vi "Backup - Acquisition Settings Dialog.vi"(8 "error in (no error)":errorcluster, 11 "Channels in":T1[](array[typedef])) -> (0 "error out":errorcluster, 3 "Channels out":T1[](array[typedef]))   [LabVIEW 2021]
uses:
  Task Cluster (with Add Remove Buttons).ctl
  DAQ/DAQ.lvlib
  Channel Cluster.ctl
panel:
  in  "Cancel Button":bool
  in  "OK Button":bool
  in  "Channel List":T2={"Add Button"=FALSE, "Remove Button"=FALSE, "DAQmx Task"="Mod3AI0-Temp", "Radio Buttons"=enum."Read"}
  # "DAQmx Global Channel"
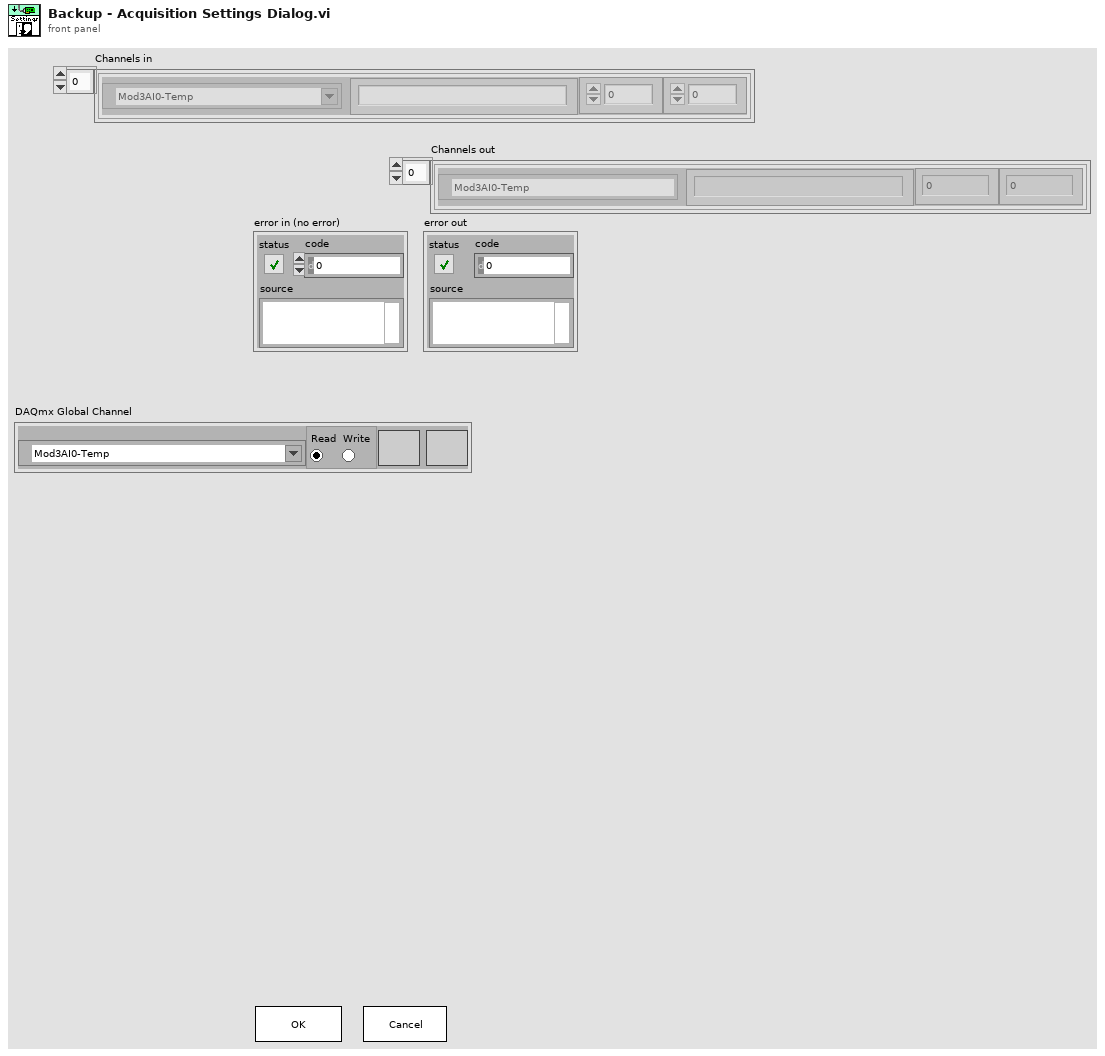
[diagram p1: front panel]
types:
  T1 = typedef "DAQ.lvlib/Channel Cluster.ctl" = cluster{"DAQmx Global Channel":refnum<k21>, "Tag Name":string, "Min Input":dbl, "Max Input":dbl}
  T2 = typedef "DAQ.lvlib/Task Cluster (with Add Remove Buttons).ctl" = cluster{"Add Button":bool, "Remove Button":bool, "DAQmx Task":refnum<k21>, "Radio Buttons":enum32{"Read", "Write"}}
  T3 = typedef "DAQ.lvlib/Channel Cluster (with Add Remove Buttons).ctl" = cluster{"Add Button":bool, "Remove Button":bool, "DAQmx Global Channel":refnum<k21>, "Tag Name":string, "Min Input":dbl, "Max Input":dbl}
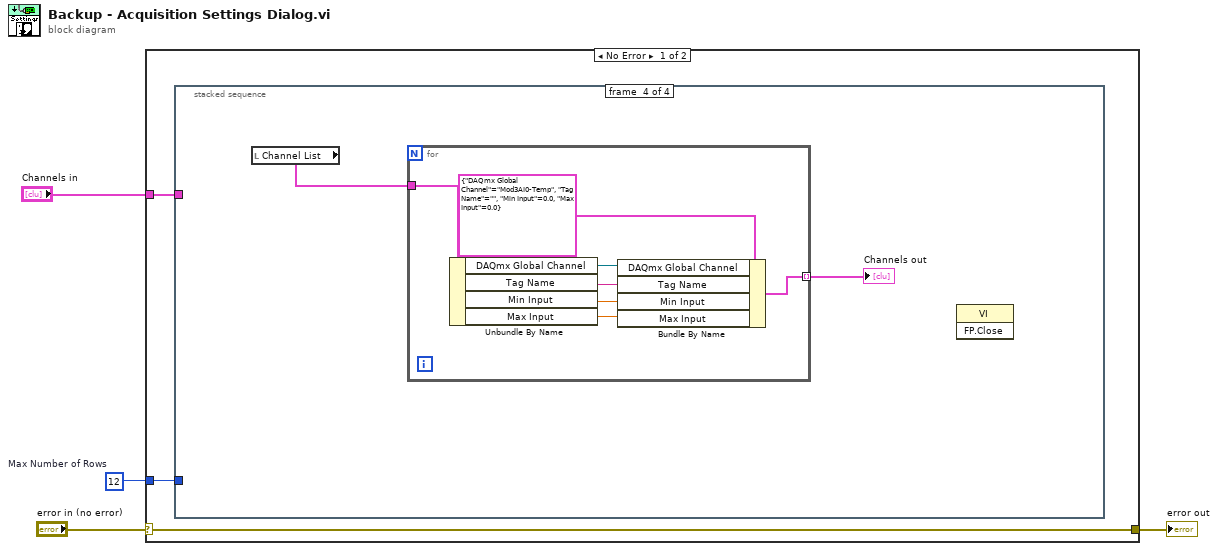
[diagram p0: block diagram]
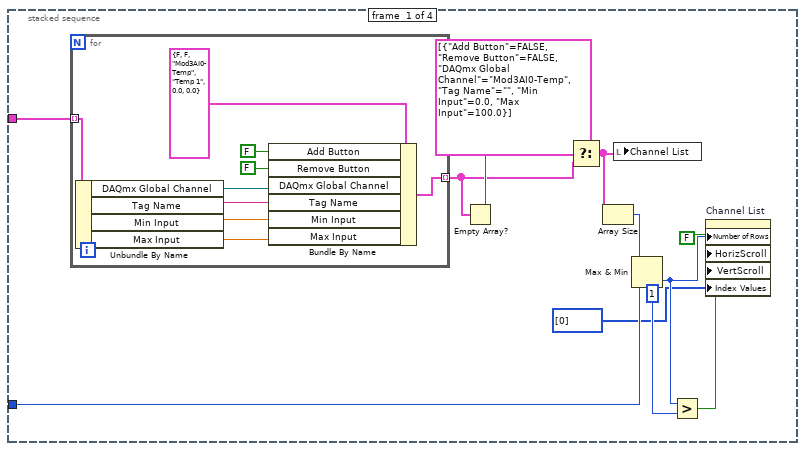
[diagram p2: hidden frame]
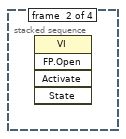
[diagram p3: hidden frame]
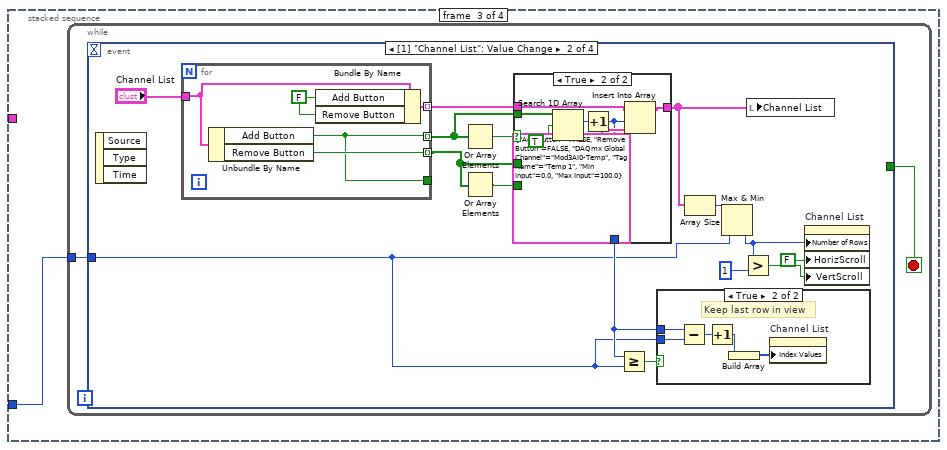
[diagram p4: hidden frame]
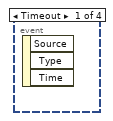
[diagram p5: hidden frame]
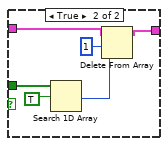
[diagram p8: hidden frame]
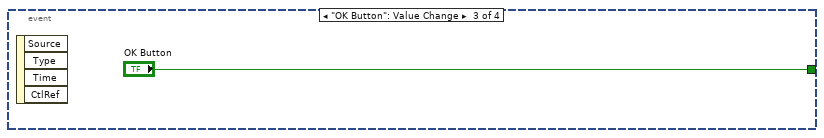
[diagram p9: hidden frame]
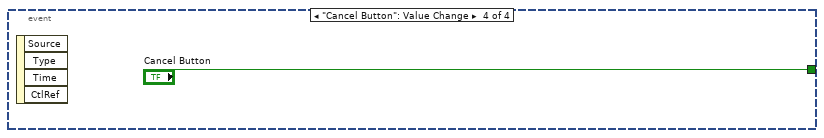
[diagram p10: hidden frame]
diagram:
  w1 = u32 12  # Max Number of Rows
  n1 = case shown="No Error" "error in (no error)" {
    selector: "error in (no error)" -> [w7 w86]
    tunnel: [w7 w86] -> w3
    tunnel: "Channels in" -> [w6 _]
    tunnel: w1 -> [w5 _]
    frame No Error {
      n2 = stacked-sequence {
        tunnel: w6 -> [w19 _ _ _]
        tunnel: w5 -> [w13 _ w29 _]
        frame #0 {
          n3 = for {
            tunnel: w19 -> [w28] mode=indexing
            tunnel: [w22] -> w16 mode=indexing
            n4 = Unbundle By Name(w28) -> ("DAQmx Global Channel"=w25:refnum<k21>, "Tag Name"=w24:string, "Min Input"=w21:dbl, "Max Input"=w20:dbl)
            n5 = Bundle By Name(cluster=T3 {"Add Button"=FALSE, "Remove Button"=FALSE, "DAQmx Global Channel"="Mod3AI0-Temp", "Tag Name"="Temp 1", "Min Input"=0.0, "Max Input"=0.0} ("DAQmx Channel Cluster"), "Add Button"=FALSE, "Remove Button"=FALSE, "DAQmx Global Channel"=w25, "Tag Name"=w24, "Min Input"=w21, "Max Input"=w20) -> (w22:T3)
          }
          n6 = Empty Array?(array=w16) -> (empty?=w18:bool)
          n7 = Select(t=T3[] [{"Add Button"=FALSE, "Remove Button"=FALSE, "DAQmx Global Channel"="Mod3AI0-Temp", "Tag Name"="", "Min Input"=0.0, "Max Input"=100.0}] ("Channel List"), s=w18, f=w16) -> (s? t:f=w15:T3[])
          n8 = Array Size(array=w15) -> (size(s)=w14:i32)
          n9 = local write "Channel List"(w15) -> ()
          n10 = Max & Min(x=w14, y=w13) -> (min(x,y)=w11:u32)  [unwired: 1 out]
          n11 = Greater?(x=w11, y=u32 1) -> (0:w9:bool)
          n12 = property on="Channel List" class="Clust"("Number of Rows"=w11, "HorizScroll"=FALSE ("Horizontal Scrollbar Visible"), "VertScroll"=w9, "Index Values"=u32[] [0]) -> ()  [unwired: 2 in, 2 out]
        }
        frame #1 {
          n13 = invoke class="VI" method="FP.Open"() -> ()  [unwired: 5 in, 5 out]
        }
        frame #2 {
          n14 = while {
            tunnel: w29 -> [w30]
            stop <- w31 stop-if-true
            n15 = event shown="[1] \"Channel List\": Value Change" {
              selector: _ -> [_ _ _ _]
              dyn-events: _ -> [_ _ _ _]
              timeout: _ -> [_ _ _ _]
              tunnel: [_ _ "OK Button" "Cancel Button"] -> w31
              tunnel: w30 -> [_ w32 _ _]
              event Timeout {
                n16 = event-data() -> ()  [unwired: 1 in, 3 out]
              }
              event Value Change {
                n17 = event-data() -> ()  [unwired: 1 in, 3 out]
                n18 = for {
                  tunnel: "Channel List" -> [w73]
                  tunnel: [w70] -> w44 mode=indexing
                  tunnel: [w74] -> w42 mode=indexing
                  tunnel: [w71] -> w43 mode=indexing
                  tunnel: [w70] -> _
                  w72 = FALSE ("Add Button")
                  n19 = Unbundle By Name(w73) -> ("Add Button"=w70:bool, "Remove Button"=w74:bool)
                  n20 = Bundle By Name(cluster=w73, "Add Button"=w72, "Remove Button"=w72) -> (w71:T2)
                }
                n21 = Or Array Elements(Boolean array=w44) -> (logical OR=w45:bool)
                n22 = Or Array Elements(Boolean array=w42) -> (logical OR=w41:bool)
                n23 = case shown="True" w45 {
                  tunnel: w44 -> [_ w69]
                  tunnel: w43 -> [w53 w67]
                  tunnel: [w52 w64] -> w40
                  tunnel: w42 -> [w55 _]
                  tunnel: w41 -> [w54 _]
                  tunnel: [_ w63] -> w33
                  frame False {
                    n24 = case shown="False" w54 {
                      tunnel: w55 -> [_ w61]
                      tunnel: w53 -> [w56 w60]
                      tunnel: [w56 w57] -> w52
                      frame False {
                      }
                      frame True {
                        n25 = Search 1D Array(1D array=w61, element=TRUE) -> (index of element=w58:i32)  [unwired: 1 in]
                        n26 = Delete From Array(array=w60, length=1, index=w58) -> (array with subset deleted=w57:T2[])  [unwired: 1 out]
                      }
                    }
                  }
                  frame True {
                    n27 = Search 1D Array(1D array=w69, element=TRUE) -> (index of element=w66:i32)  [unwired: 1 in]
                    n28 = Increment(x=w66) -> (x+1=w63:i32)
                    n29 = Insert Into Array(array=w67, index=w63, new element=T3 {"Add Button"=FALSE, "Remove Button"=FALSE, "DAQmx Global Channel"="Mod3AI0-Temp", "Tag Name"="Temp 1", "Min Input"=0.0, "Max Input"=100.0} ("new element/subarray")) -> (w64:T2[])
                  }
                }
                n30 = Greater Or Equal?(x=w33, y=w32) -> (x >= y?=w34:bool)
                n31 = case shown="True" w34 {
                  tunnel: w33 -> [_ w51]
                  tunnel: w32 -> [_ w50]
                  frame False {
                  }
                  frame True {
                    # "Keep last row in view"
                    n32 = Subtract(x=w51, y=w50) -> (x-y=w49:u32)
                    n33 = Increment(x=w49) -> (x+1=w47:u32)
                    n34 = Build Array(w47) -> (w48:u32[])
                    n35 = property on="Channel List" class="Clust"("Index Values"=w48) -> ()  [unwired: 2 in, 2 out]
                  }
                }
                n36 = Array Size(array=w40) -> (size(s)=w39:i32)
                n37 = Max & Min(x=w39, y=w32) -> (min(x,y)=w36:u32)  [unwired: 1 out]
                n38 = Greater?(x=w36, y=u32 1) -> (0:w35:bool)
                n39 = local write "Channel List"(w40) -> ()
                n40 = property on="Channel List" class="Clust"("Number of Rows"=w36, "HorizScroll"=FALSE ("Horizontal Scrollbar Visible"), "VertScroll"=w35) -> ()  [unwired: 2 in, 2 out]
              }
              event "OK Button": Value Change {
                n41 = event-data() -> ()  [unwired: 1 in, 4 out]
              }
              event "Cancel Button": Value Change {
                n42 = event-data() -> ()  [unwired: 1 in, 4 out]
              }
            }
          }
        }
        frame #3 {
          n43 = local read "Channel List"() -> (w78:T2)
          n44 = for {
            tunnel: w78 -> [w85]
            tunnel: [w81] -> w77 mode=indexing
            n45 = Unbundle By Name(w85) -> ("DAQmx Global Channel"=w83:refnum<k21>, "Tag Name"=w82:string, "Min Input"=w80:dbl, "Max Input"=w79:dbl)
            n46 = Bundle By Name(cluster=T1 {"DAQmx Global Channel"="Mod3AI0-Temp", "Tag Name"="", "Min Input"=0.0, "Max Input"=0.0} ("DAQmx Channel Cluster"), "DAQmx Global Channel"=w83, "Tag Name"=w82, "Min Input"=w80, "Max Input"=w79) -> (w81:T1)
          }
          "Channels out" <- w77
          n47 = invoke class="VI" method="FP.Close"() -> ()  [unwired: 3 in, 3 out]
        }
      }
    }
    frame Error {
    }
  }
  "error out" <- w3
